vi "Code Report CLI.vi"(11 "Command Line Args":string[](array[string])=["SearchPath=\"..\\..\\Source\\\"", "ReportPath=\"..\\..\\CodeReport.xml\"", "Recursive=true", "ListParams=false"]) -> (2 "Return Message":string="No Error", 3 "Return Code":i32)   [LabVIEW 2016]
uses:
  Command Line Arguments.ctl
  <vilib>/Utility/error.llb/DialogType.ctl
  <vilib>/ni/Simple XML/_polymorphics/Create Tag - Root.vi
  <vilib>/ni/Simple XML/_polymorphics/Create Tag - Child.vi
  <vilib>/ni/Simple XML/_polymorphics/Create Tag - Child with Text.vi
  <vilib>/xml/Close Reference(Node).vi
  <vilib>/xml/NI_XML.lvlib
  <vilib>/ni/Simple XML/Simple XML.lvlib
  <resource>/objmgr/DOMUserDefRef.rc
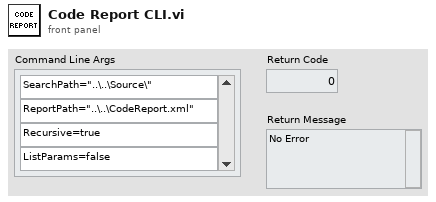
[diagram p1: front panel]
types:
  T1 = typedef "DialogType.ctl" = u16
  T2 = typedef "Command Line Arguments.ctl" = cluster{"Search Path":path, "Report Path":path, "Recursive Search?":bool, "List Parameters?":bool}
  T3 = cluster{string, "filename without extension":string, refnum<vi>}
  T4 = cluster{string, "filename without extension":string, refnum<vi>}[]
  T5 = enum32{"invalid VI type", "Standard VI", "Control VI", "Global VI", "Polymorphic VI", "Configuration VI", "SubSystem", "Facade VI", "Method VI", "Statechart Diagram VI"}
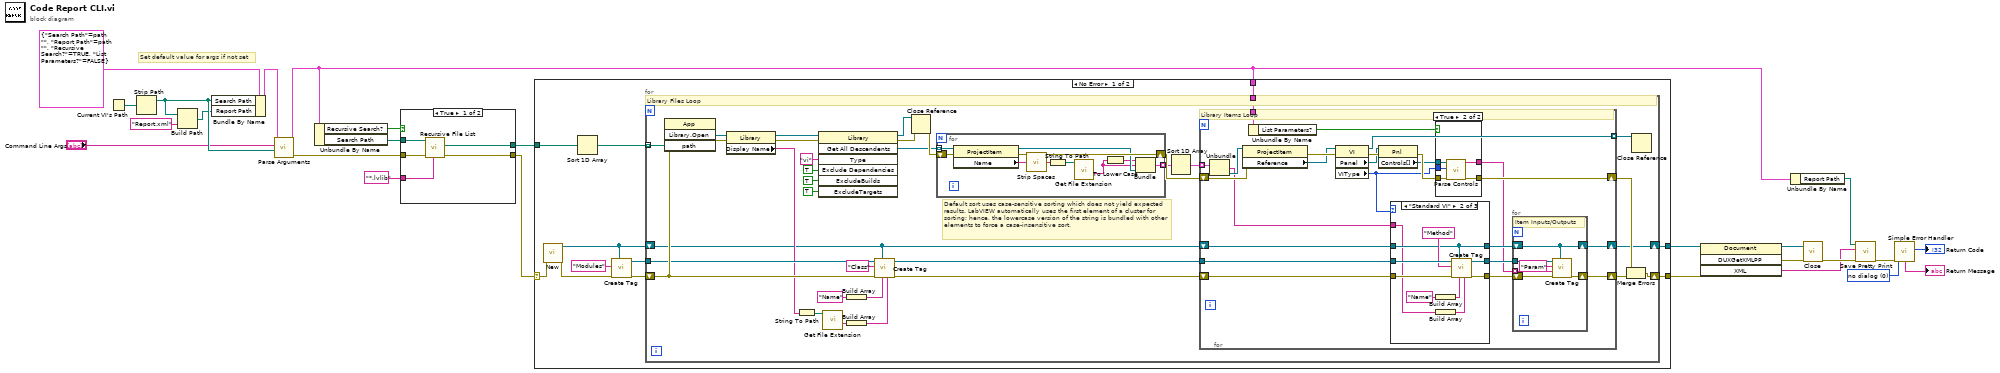
[diagram p0: block diagram]
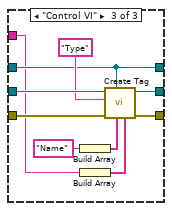
[diagram p4: hidden frame]
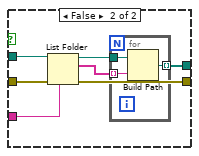
[diagram p6: hidden frame]
diagram:
  w4 = T1 0 items=["no dialog", "OK message", "continue or stop message", "OK message + warnings", "continue/stop + warnings"] ("type of dialog (OK msg:1)")
  # "Set default value for args if not set"
  n1 = Current VI's Path() -> (path=w10:path)
  n2 = Strip Path(path=w10) -> (stripped path=w19:path)  [unwired: 1 out]
  n3 = Build Path(base path=w19, name or relative path="Report.xml") -> (appended path=w7:path)
  n4 = Bundle By Name(cluster=T2 {"Search Path"=path "", "Report Path"=path "", "Recursive Search?"=TRUE, "List Parameters?"=FALSE} ("Default Values"), "Search Path"=w19, "Report Path"=w7) -> (w8:T2)
  n5 = call "Parse Arguments.vi"("Working Directory"=w19, "Command Line Args"="Command Line Args", "Parameters in"=w8) -> ("error constant"=w25:errorcluster, "Parameters out"=w5:T2)  [unwired: 7 in]
  n6 = Unbundle By Name(w5) -> ("Recursive Search?"=w12:bool, "Search Path"=w16:path)
  n7 = case shown="True" w12 {
    tunnel: "*.lvlib" ("pattern") -> [w28 w35]
    tunnel: w16 -> [w27 w34]
    tunnel: w25 -> [w30 w37]
    tunnel: [w29 w36] -> w20
    tunnel: [w26 w31] -> w1
    frame True {
      n8 = call <vilib>:"Recursive File List.vi"("pattern"=w28, "error in (no error)"=w30, "Folder Path"=w27) -> ("error out"=w29:errorcluster, "All Files in Dir"=w26:path[])  [unwired: 4 in, 3 out]
    }
    frame False {
      n9 = List Folder(path=w34, pattern=w35, error in=w37) -> (path out=w33:path, filenames=w32:string[], error out=w36:errorcluster)  [unwired: 1 in, 1 out]
      n10 = for {
        tunnel: w33 -> [w40]
        tunnel: w32 -> [w39] mode=indexing
        tunnel: [w38] -> w31 mode=indexing
        n11 = Build Path(base path=w40, name or relative path=w39) -> (appended path=w38:path)
      }
    }
  }
  n12 = case shown="No Error" w20 {
    selector: w20 -> [w49 w155]
    tunnel: [w51 w155] -> w22
    tunnel: [w47 _] -> w11
    tunnel: w5 -> [w46 _]
    tunnel: w1 -> [w42 _]
    frame No Error {
      n13 = call <vilib>:"New.vi"("error in (no error)"=w49) -> ("error out"=w50:errorcluster, "DOM document out"=w43:refnum<k20>)  [unwired: 7 in]
      n14 = Sort 1D Array(array=w42) -> (sorted array=w41:path[])
      n15 = call-poly <vilib>:"Create Tag.vi"("DOM document reference"=w43, "error in (no error)"=w50, "Tag Name"="Modules") -> ("error out"=w48:errorcluster, "Element reference"=w44:refnum<k20>)  [unwired: 7 in]
      n16 = for {
        tunnel: w41 -> [w75] mode=indexing
        tunnel: w44 -> [w73]
        shift-right: [w56] -> w47
        shift-left: w43 -> [w57]
        shift-right: [w77] -> w51
        shift-left: w48 -> [w83]
        tunnel: w46 -> [w52]
        # "Default sort uses case-sensitive sorting which does not yield expected results. LabVIEW automatically uses the first element of a cluster for sorting; hence, the lowercase version of the string is bundled with other elements to force a case-insensitive sort."
        # "Library Files Loop"
        n17 = invoke class="App" method="Library.Open"(error in=w83, "path"=w75) -> (error out=w84:errorcluster, "Open Library"=w74:refnum<vi>)  [unwired: 2 in, 2 out]
        n18 = property class="Library"(reference=w74, error in=w84) -> (reference out=w64:refnum<vi>, error out=w85:errorcluster, "Display Name"=w70:string)
        n19 = String To Path(string=w70) -> (path=w67:path)
        n20 = invoke class="Library" method="Get All Descendents"(reference=w64, error in=w85, "Type"="vi", "Exclude Dependencies"=TRUE ("ExcludeDependencies"), "ExcludeBuilds"=TRUE, "ExcludeTargets"=TRUE) -> (reference out=w60:refnum<vi>, error out=w82:errorcluster, "All Descendents"=w54:refnum<vi>[])  [unwired: 1 in, 4 out]
        n21 = call <vilib>:"Get File Extension.vi"("file"=w67) -> ("filename without extension"=w66:string)  [unwired: 6 in, 4 out]
        n22 = Build Array("Name" ("Tag Name")) -> (w68:string[])
        n23 = Build Array(w66) -> (w71:string[])
        n24 = call-poly <vilib>:"Create Tag.vi"("Attr Values"=w71, "Attr Names"=w68, "DOM Document reference"=w57, "error in (no error)"=w83, "Tag Name"="Class", "Parent Element reference"=w73) -> ("error out"=w81:errorcluster, "Child Element reference"=w58:refnum<k20>)  [unwired: 4 in]
        n25 = Close Reference(reference=w60, error in (no error)=w82) -> (error out=w79:errorcluster)
        n26 = for {
          tunnel: w54 -> [w93] mode=indexing
          tunnel: [w91] -> w55 mode=indexing
          shift-right: [w94] -> w78
          shift-left: w79 -> [w95]
          n27 = property class="ProjectItem"(reference=w93, error in=w95) -> (reference out=w92:refnum<vi>, error out=w94:errorcluster, "Name"=w88:string)
          n28 = call "Strip Spaces.vi"("String In"=w88) -> ("result string"=w90:string)  [unwired: 14 in]
          n29 = String To Path(string=w90) -> (path=w89:path)
          n30 = call <vilib>:"Get File Extension.vi"("file"=w89) -> ("filename without extension"=w87:string)  [unwired: 6 in, 4 out]
          n31 = To Lower Case(string=w87) -> (all lower case string=w86:string)
          n32 = Bundle(w86, "filename without extension"=w87, w92) -> (w91:T3)  [unwired: 1 in]
        }
        n33 = Sort 1D Array(array=w55) -> (sorted array=w53:T4)
        n34 = for {
          tunnel: [w110] -> w59 mode=indexing
          tunnel: w58 -> [w108]
          shift-right: [w101] -> w56
          shift-left: w57 -> [w107]
          shift-right: [w114] -> w80
          shift-left: w81 -> [w117]
          tunnel: w53 -> [w106] mode=indexing
          shift-right: [w113] -> w76
          shift-left: w78 -> [w112]
          tunnel: w52 -> [w100]
          # "Library Items Loop"
          n35 = Unbundle(w106) -> ("filename without extension"=w96:string, w97:refnum<vi>)  [unwired: 1 out]
          n36 = property class="ProjectItem"(reference=w97, error in=w112) -> (error out=w119:errorcluster, "Reference"=w111:refnum<vi>)  [unwired: 1 out]
          n37 = Unbundle By Name(w100) -> ("List Parameters?"=w99:bool)
          n38 = property class="VI"(reference=w111, error in=w119) -> (reference out=w110:refnum<vi>, error out=w118:errorcluster, "Panel"=w109:refnum<vi>, "VIType"=w98:T5)
          n39 = property class="Pnl"(reference=w109, error in=w118) -> (error out=w116:errorcluster, "Controls[]"=w105:refnum<vi>[])  [unwired: 1 out]
          n40 = case shown="\"Standard VI\"" w98 {
            tunnel: w117 -> [w134 w144 w154]
            tunnel: w108 -> [w132 w142 w152]
            tunnel: w96 -> [_ w136 w146]
            tunnel: [w134 w143 w153] -> w115
            tunnel: w107 -> [w133 w140 w150]
            tunnel: [w133 w140 w150] -> w103
            tunnel: [w132 w139 w149] -> w104
            frame Default {
            }
            frame "Standard VI" {
              n41 = Build Array("Name" ("Tag Name")) -> (w137:string[])
              n42 = Build Array(w136) -> (w135:string[])
              n43 = call-poly <vilib>:"Create Tag.vi"("Attr Values"=w135, "Attr Names"=w137, "DOM Document reference"=w140, "error in (no error)"=w144, "Tag Name"="Method", "Parent Element reference"=w142) -> ("error out"=w143:errorcluster, "Child Element reference"=w139:refnum<k20>)  [unwired: 4 in]
            }
            frame "Control VI" {
              n44 = Build Array("Name" ("Tag Name")) -> (w147:string[])
              n45 = Build Array(w146) -> (w145:string[])
              n46 = call-poly <vilib>:"Create Tag.vi"("Attr Values"=w145, "Attr Names"=w147, "DOM Document reference"=w150, "error in (no error)"=w154, "Tag Name"="Type", "Parent Element reference"=w152) -> ("error out"=w153:errorcluster, "Child Element reference"=w149:refnum<k20>)  [unwired: 4 in]
            }
          }
          n47 = case shown="True" w99 {
            tunnel: w105 -> [_ w123]
            tunnel: w116 -> [w120 w125]
            tunnel: [_ w122] -> w102
            tunnel: [w120 w124] -> w113
            tunnel: w98 -> [_ w121]
            frame False {
            }
            frame True {
              n48 = call "Parse Controls.vi"("error in (no error)"=w125, "VI Type"=w121, "Controls[]"=w123) -> ("error out"=w124:errorcluster, "Control Names"=w122:string[])  [unwired: 7 in]
            }
          }
          n49 = for {
            tunnel: w104 -> [w129]
            shift-right: [w130] -> w114
            shift-left: w115 -> [w131]
            tunnel: w102 -> [w128] mode=indexing
            shift-right: [w126] -> w101
            shift-left: w103 -> [w126]
            # "Item Inputs/Outputs"
            n50 = call-poly <vilib>:"Create Tag.vi"("DOM document reference"=w126, "error in (no error)"=w131, "Text Data"=w128, "Tag Name"="Param", "Parent Element reference"=w129) -> ("error out"=w130:errorcluster)  [unwired: 5 in, 1 out]
          }
        }
        n51 = Merge Errors(w76, w80) -> (w77:errorcluster)
        n52 = Close Reference(reference=w59) -> ()  [unwired: 1 in, 1 out]
      }
    }
    frame Error {
    }
  }
  n53 = invoke class="Document" method="DUXGetXMLPP"(reference=w11, error in=w22) -> (reference out=w15:refnum<k20>, error out=w23:errorcluster, "XML"=w14:string)  [unwired: 2 in, 1 out]
  n54 = Unbundle By Name(w5) -> ("Report Path"=w13:path)
  n55 = call-poly <vilib>:"Close.vi"("error in (no error)"=w23, "node"=w15) -> ("error out"=w24:errorcluster)  [unwired: 7 in]
  n56 = call <vilib>:"Save Pretty Print.vi"("error in (no error)"=w24, "Pretty XML String"=w14, "XML file path"=w13) -> ("error out"=w21:errorcluster)  [unwired: 7 in, 1 out]
  n57 = call <vilib>:"Simple Error Handler.vi"("type of dialog (OK msg:1)"=w4, "error in (no error)"=w21) -> ("code out"=→"Return Code":i32, "message"=→"Return Message":string)  [unwired: 3 in, 3 out]
